vi "FL Set Membership Function (Fuzzy System).vi"(0 "fuzzy system in":T2 {"user MF interpolating polynomials"."coa_x(y) coeff" format="%.4g"; "user MF interpolating polynomials"."Area(y) coeff" format="%.4g"; "user MF interpolating polynomials"."X(y) coeff" format="%.4g"; "user MF interpolating polynomials"."Y(x) coeff" format="%.4g"; "user MF interpolating polynomials"."Y" format="%.4g"; "user MF interpolating polynomials"."X" format="%.4g"; "defuzzification method" items=["Center of Area", "Modified Center of Area", "Center of Sums", "Center of Maximum", "Mean of Maximum"]; "rules"."consequents"."Var Index" min=0; "rules"."consequents"."Cond" items=["=", "!="]; "rules"."consequents"."MF Index" min=0; "rules"."antecedents"."Var Index" min=0; "rules"."antecedents"."Cond" items=["=", "!="]; "rules"."antecedents"."MF Index" min=0; "rules"."consequent implication" items=["Minimum", "Product"]; "rules"."antecedent connective" items=["AND (Minimum)", "AND (Product)", "OR (Maximum)", "OR (Probabilistic)"]; "output variables"."MFs"."shape" items=["Triangle", "Trapezoid", "Singleton", "Sigmoid", "Gaussian", "User-Defined"]; "input variables"."MFs"."shape" items=["Triangle", "Trapezoid", "Singleton", "Sigmoid", "Gaussian", "User-Defined"]}, 1 "input/output":enum16{"Input", "Output"}(ring), 2 "variable index":i32, 3 "membership function index":i32, 5 "name":string, 7 "shape":T1 items=["Triangle", "Trapezoid", "Singleton", "Sigmoid", "Gaussian", "User-Defined"], 9 "points":dbl[](array[numeric]), 11 "error in (no error)":errorcluster, 12 "color":u32(colorbox)=16777215, 13 "user-defined shape index":i32) -> (4 "fuzzy system out":T2 {"user MF interpolating polynomials"."coa_x(y) coeff" format="%.4g"; "user MF interpolating polynomials"."Area(y) coeff" format="%.4g"; "user MF interpolating polynomials"."X(y) coeff" format="%.4g"; "user MF interpolating polynomials"."Y(x) coeff" format="%.4g"; "user MF interpolating polynomials"."Y" format="%.4g"; "user MF interpolating polynomials"."X" format="%.4g"; "defuzzification method" items=["Center of Area", "Modified Center of Area", "Center of Sums", "Center of Maximum", "Mean of Maximum"]; "rules"."consequents"."Var Index" min=0; "rules"."consequents"."Cond" items=["=", "!="]; "rules"."consequents"."MF Index" min=0; "rules"."antecedents"."Var Index" min=0; "rules"."antecedents"."Cond" items=["=", "!="]; "rules"."antecedents"."MF Index" min=0; "rules"."consequent implication" items=["Minimum", "Product"]; "rules"."antecedent connective" items=["AND (Minimum)", "AND (Product)", "OR (Maximum)", "OR (Probabilistic)"]; "output variables"."MFs"."shape" items=["Triangle", "Trapezoid", "Singleton", "Sigmoid", "Gaussian", "User-Defined"]; "input variables"."MFs"."shape" items=["Triangle", "Trapezoid", "Singleton", "Sigmoid", "Gaussian", "User-Defined"]}, 15 "error out":errorcluster)   [LabVIEW 2013, in "NI_Fuzzy_Logic_API.lvlib"]
doc: "Modifies the shape, color, or points of a membership function for a linguistic variable. You can modify a membership function from a fuzzy system or from an array of membership functions. The data type you wire to the <B>fuzzy system in</B> input determines the polymorphic instance to use."
uses:
  <vilib>/addons/Fuzzy Logic/NI_Fuzzy_Logic_API.lvlib
  <vilib>/addons/Fuzzy Logic/TypeDefs/FL System.ctl
  <vilib>/addons/Fuzzy Logic/TypeDefs/FL Variable.ctl
  <vilib>/addons/Fuzzy Logic/TypeDefs/FL Membership Function.ctl
  <vilib>/addons/Fuzzy Logic/TypeDefs/FL Membership Function Shape.ctl
  <vilib>/addons/Fuzzy Logic/TypeDefs/FL Rule.ctl
  <vilib>/addons/Fuzzy Logic/TypeDefs/FL Antecedent.ctl
  <vilib>/addons/Fuzzy Logic/TypeDefs/FL Modifier.ctl
  <vilib>/addons/Fuzzy Logic/TypeDefs/FL Antecedent Connective.ctl
  <vilib>/addons/Fuzzy Logic/TypeDefs/FL Consequent.ctl
  <vilib>/addons/Fuzzy Logic/TypeDefs/FL Consequent Implication.ctl
  <vilib>/addons/Fuzzy Logic/TypeDefs/FL Defuzzification.ctl
  <vilib>/addons/Fuzzy Logic/TypeDefs/FL Interpolating polynomials.ctl
panel:
  # "IF"
  # "THEN"
  # "IF"
  # "THEN"
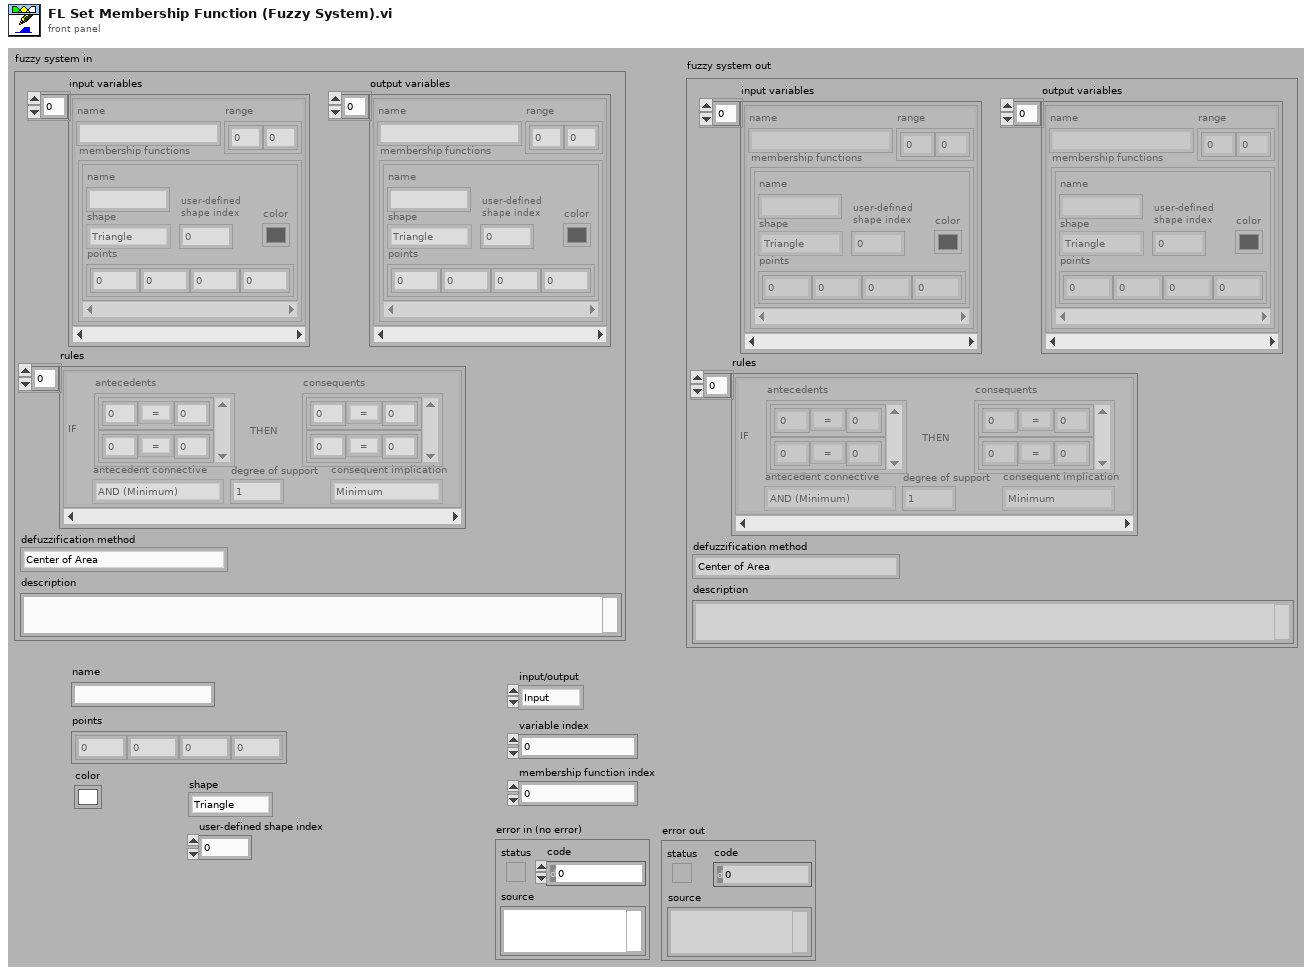
[diagram p1: front panel]
types:
  T1 = typedef "NI_Fuzzy_Logic_API.lvlib/FL Membership Function Shape.ctl" = u16
  T2 = typedef "NI_Fuzzy_Logic_API.lvlib/FL System.ctl" = cluster{"input variables":T3[], "output variables":T3[], "rules":T5[], "defuzzification method":T11, "description":string, "user MF interpolating polynomials":T12[]}
  T3 = typedef "NI_Fuzzy_Logic_API.lvlib/FL Variable.ctl" = cluster{"name":string, "range":dbl[], "MFs":T4[]}
  T4 = typedef "NI_Fuzzy_Logic_API.lvlib/FL Membership Function.ctl" = cluster{"name":string, "shape":T1, "points":dbl[], "color":u32, "user-defined shape index":i32}
  T5 = typedef "NI_Fuzzy_Logic_API.lvlib/FL Rule.ctl" = cluster{"antecedents":T6[], "antecedent connective":T8, "consequents":T9[], "consequent implication":T10, "degree of support":dbl}
  T6 = typedef "NI_Fuzzy_Logic_API.lvlib/FL Antecedent.ctl" = cluster{"Var Index":i32, "MF Index":i32, "Cond":T7}
  T7 = typedef "NI_Fuzzy_Logic_API.lvlib/FL Modifier.ctl" = u16
  T8 = typedef "NI_Fuzzy_Logic_API.lvlib/FL Antecedent Connective.ctl" = u16
  T9 = typedef "NI_Fuzzy_Logic_API.lvlib/FL Consequent.ctl" = cluster{"Var Index":i32, "MF Index":i32, "Cond":T7}
  T10 = typedef "NI_Fuzzy_Logic_API.lvlib/FL Consequent Implication.ctl" = u16
  T11 = typedef "NI_Fuzzy_Logic_API.lvlib/FL Defuzzification.ctl" = u16
  T12 = typedef "NI_Fuzzy_Logic_API.lvlib/FL Interpolating polynomials.ctl" = cluster{"X":dbl[], "Y":dbl[], "Y(x) coeff":dbl[][], "X(y) coeff":dbl[][], "Area(y) coeff":dbl[][], "coa_x(y) coeff":dbl[][]}
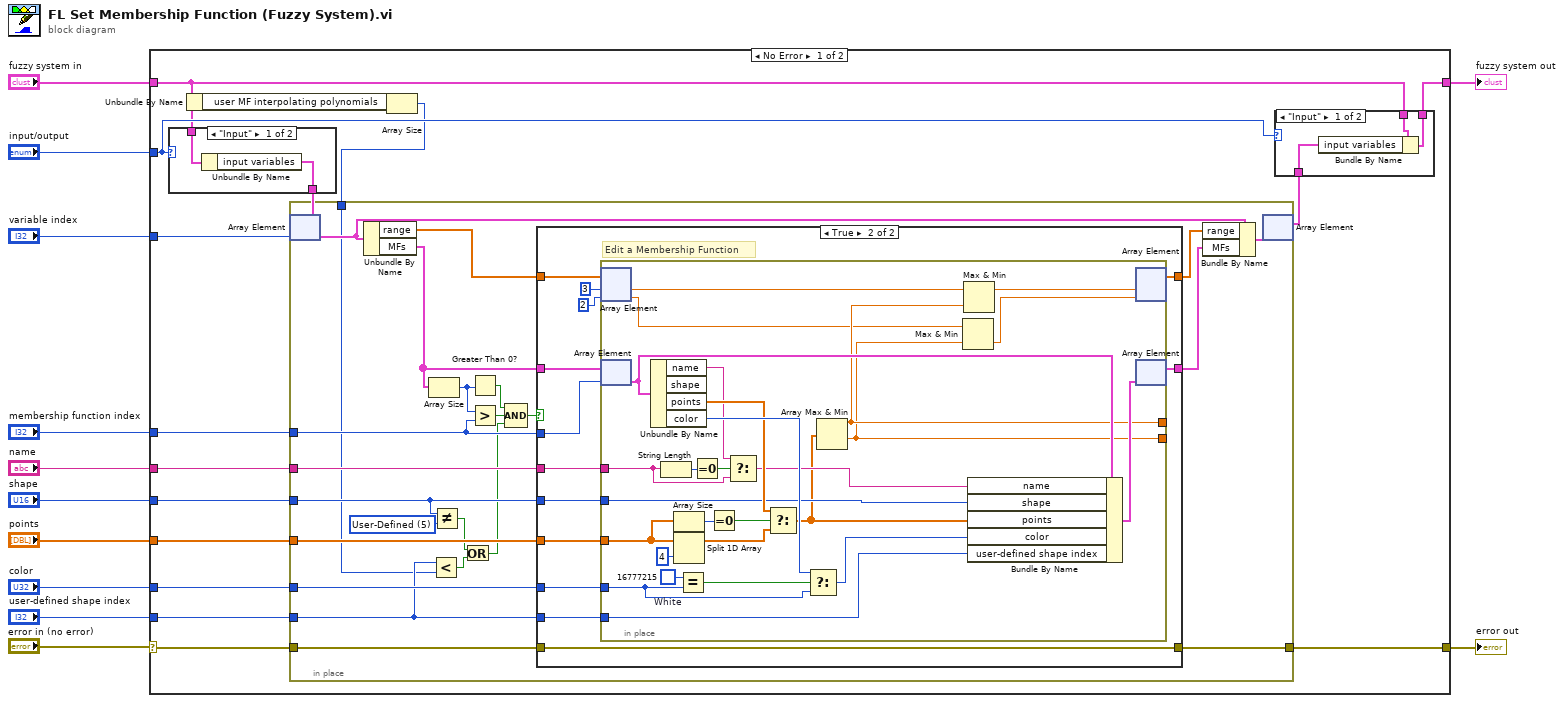
[diagram p0: block diagram]
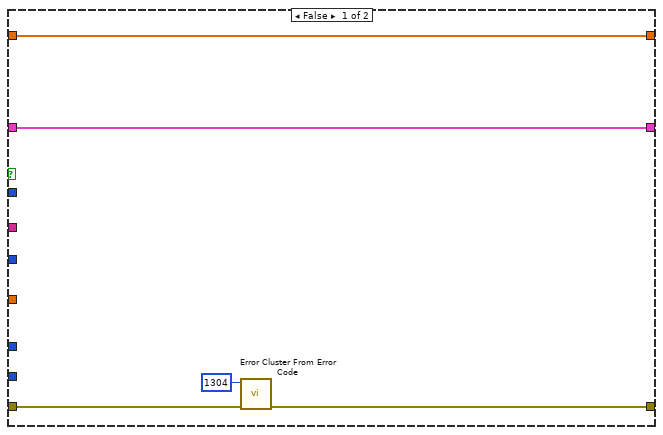
[diagram p2: hidden frame]
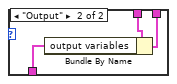
[diagram p3: hidden frame]
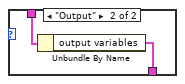
[diagram p4: hidden frame]
diagram:
  n1 = case shown="No Error" "error in (no error)" {
    selector: "error in (no error)" -> [w18 w107]
    tunnel: "fuzzy system in" -> [w15 w108]
    tunnel: [w28 w108] -> w11
    tunnel: "input/output" -> [w27 _]
    tunnel: "variable index" -> [w24 _]
    tunnel: "membership function index" -> [w23 _]
    tunnel: "name" -> [w22 _]
    tunnel: "shape" -> [w21 _]
    tunnel: "color" -> [w20 _]
    tunnel: "points" -> [w19 _]
    tunnel: [w17 w107] -> w2
    tunnel: "user-defined shape index" -> [w16 _]
    frame No Error {
      n2 = case shown="\"Input\"" w27 {
        tunnel: [w104 w105] -> w26
        tunnel: w15 -> [w103 w106]
        frame "Input" {
          n3 = Unbundle By Name(w103) -> ("input variables"=w104:T3[])
        }
        frame "Output" {
          n4 = Unbundle By Name(w106) -> ("output variables"=w105:T3[])
        }
      }
      n5 = Unbundle By Name(w15) -> ("user MF interpolating polynomials"=w14:T12[])
      n6 = Array Size(array=w14) -> (size(s)=w13:i32)
      n7 = in-place {
        in-place-border: w23 -> [w44]
        in-place-border: w22 -> [w43]
        in-place-border: w21 -> [w35]
        in-place-border: w19 -> [w41]
        in-place-border: w20 -> [w42]
        in-place-border: w18 -> [w39]
        in-place-border: [w38] -> w17
        in-place-border: w16 -> [w33]
        in-place-border: w13 -> [w32]
        w34 = T1 5 items=["Triangle", "Trapezoid", "Singleton", "Sigmoid", "Gaussian", "User-Defined"] ("y")
        n8 = in-place-array #1(w26, w24) -> (w46:T3)
        n9 = Unbundle By Name(w46) -> ("range"=w37:dbl[], "MFs"=w40:T4[])
        n10 = Array Size(array=w40) -> (size(s)=w49:i32)
        n11 = Less?(x=w33, y=w32) -> (x < y?=w31:bool)
        n12 = Not Equal?(x=w35, y=w34) -> (x != y?=w30:bool)
        n13 = Or(x=w30, y=w31) -> (x .or. y?=w29:bool)
        n14 = Greater Than 0?(x=w49) -> (x > 0?=w48:bool)
        n15 = Greater?(x=w49, y=w44) -> (0:w50:bool)
        n16 = Compound Arithmetic op=AND(w48, w50, w29) -> (w47:bool)
        n17 = case shown="True" w47 {
          tunnel: w44 -> [_ w67]
          tunnel: [w56 w68] -> w51
          tunnel: w40 -> [w56 w69]
          tunnel: w43 -> [_ w66]
          tunnel: w42 -> [_ w64]
          tunnel: w41 -> [_ w65]
          tunnel: w35 -> [_ w63]
          tunnel: w39 -> [w55 w62]
          tunnel: [w53 w62] -> w38
          tunnel: w37 -> [w52 w61]
          tunnel: [w52 w58] -> w36
          tunnel: w33 -> [_ w57]
          frame False {
            n18 = call <vilib>:"Error Cluster From Error Code.vi"("error in (no error)"=w55, "error code (0)"=1304) -> ("error out"=w53:errorcluster)  [unwired: 1 in, 6 out]
          }
          frame True {
            # "Edit a Membership Function"
            n19 = in-place {
              in-place-border: w65 -> [w84]
              in-place-border: w66 -> [w86]
              in-place-border: w64 -> [w85]
              in-place-border: w63 -> [w73]
              in-place-border: [w79] -> _
              in-place-border: [w78] -> _
              in-place-border: w57 -> [w70]
              w92 = u32 16777215  # White
              n20 = in-place-array #2(w61, 3, 2) -> (w80:dbl, w77:dbl)
              n21 = in-place-array #3(w69, w67) -> (w81:T4)
              n22 = Unbundle By Name(w81) -> ("name"=w90:string, "points"=w94:dbl[], "color"=w95:u32)  [unwired: 1 out]
              n23 = String Length(string=w86) -> (length=w89:i32)
              n24 = Array Size(array=w84) -> (size(s)=w96:i32)
              n25 = Split 1D Array(array=w84, index=4) -> (first subarray=w82:dbl[])  [unwired: 1 out]
              n26 = Equal?(x=w92, y=w85) -> (x = y?=w93:bool)
              n27 = Equal To 0?(x=w89) -> (x = 0?=w88:bool)
              n28 = Equal To 0?(x=w96) -> (x = 0?=w91:bool)
              n29 = Select(t=w90, s=w88, f=w86) -> (s? t:f=w74:string)
              n30 = Select(t=w94, s=w91, f=w82) -> (s? t:f=w72:dbl[])
              n31 = Select(t=w95, s=w93, f=w85) -> (s? t:f=w71:u32)
              n32 = Array Max & Min(array=w72) -> (max value=w79:dbl, min value=w78:dbl)  [unwired: 2 out]
              n33 = Max & Min(x=w77, y=w78) -> (min(x,y)=w76:dbl)  [unwired: 1 out]
              n34 = Max & Min(x=w80, y=w79) -> (max(x,y)=w75:dbl)  [unwired: 1 out]
              n35 = Bundle By Name(cluster=w81, "name"=w74, "shape"=w73, "points"=w72, "color"=w71, "user-defined shape index"=w70) -> (w87:T4)
              n36 = in-place-array #2(w75, w76) -> (w58:dbl[])  [unwired: 2 out]
              n37 = in-place-array #3(w87) -> (w68:T4[])  [unwired: 1 out]
            }
          }
        }
        n38 = Bundle By Name(cluster=w46, "range"=w36, "MFs"=w51) -> (w45:T3)
        n39 = in-place-array #1(w45) -> (w25:T3[])  [unwired: 1 out]
      }
      n40 = case shown="\"Input\"" w27 {
        tunnel: w15 -> [w99 w102]
        tunnel: [w98 w101] -> w28
        tunnel: w25 -> [w97 w100]
        frame "Input" {
          n41 = Bundle By Name(cluster=w99, "input variables"=w97) -> (w98:T2)
        }
        frame "Output" {
          n42 = Bundle By Name(cluster=w102, "output variables"=w100) -> (w101:T2)
        }
      }
    }
    frame Error {
    }
  }
  "fuzzy system out" <- w11
  "error out" <- w2
